vi "Day 23-Recurse Possible Moves.vi"(10 "Energy in":i32, 11 "State in":map{T1, T2[]}(c390)) -> (2 "Energy out":i32, 3 "State out":map{T1, T2[]}(c390))   [LabVIEW 2021]
uses:
  Amphipod Enum.ctl
  3c6be11d-fb2c-47dd-b0ed-e6924b9f2e6b.vi
  Zone Enum.ctl
  Hallway Positions Enum.ctl
  Room Enum.ctl
  Position Cluster.ctl
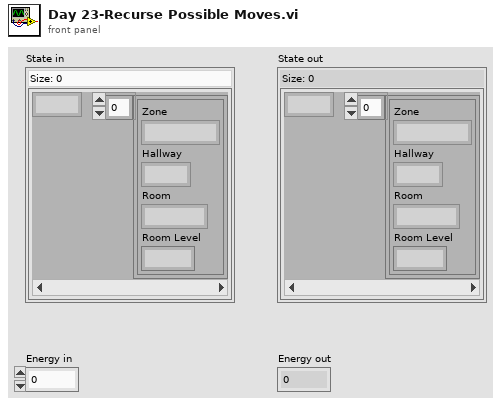
[diagram p1: front panel]
types:
  T1 = typedef "Amphipod Enum.ctl" = enum16{"A", "B", "C", "D"}
  T2 = typedef "Position Cluster.ctl" = cluster{"Zone":T3, "Hallway":T4, "Room":T5, "Room Level":i32}
  T3 = typedef "Zone Enum.ctl" = enum16{"Hallway", "Room"}
  T4 = typedef "Hallway Positions Enum.ctl" = enum16{"H1", "H2", "D3", "H4", "D5", "H6", "D7", "H8", "D9", "H10", "H11"}
  T5 = typedef "Room Enum.ctl" = enum16{"Room A", "Room B", "Room C", "Room D"}
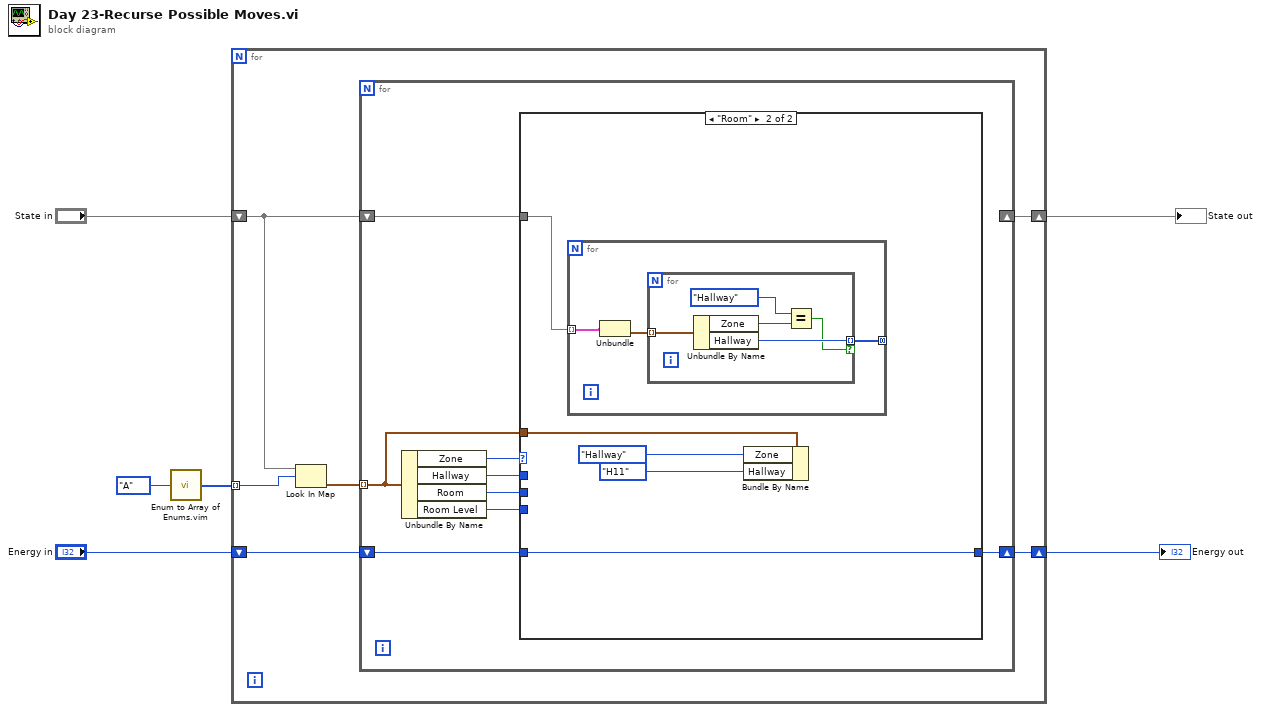
[diagram p0: block diagram]
diagram:
  n1 = call "Enum to Array of Enums.vim"("enum"=Amphipod_Enum."A" ("Amphipod Enum")) -> ("array of enums"=w1:T1[])
  n2 = for {
    tunnel: w1 -> [w12] mode=indexing
    shift-right: [w9] -> w6
    shift-left: "Energy in" -> [w10]
    shift-right: [w7] -> w3
    shift-left: "State in" -> [w8]
    n3 = Look In Map(map=w8, key=w12) -> (value=w11:T2[])  [unwired: 1 in, 1 out]
    n4 = for {
      tunnel: w11 -> [w13] mode=indexing
      shift-right: [w15] -> w9
      shift-left: w10 -> [w16]
      shift-right: [_] -> w7
      shift-left: w8 -> [w14]
      n5 = Unbundle By Name(w13) -> ("Zone"=w20:T3, "Hallway"=w19:T4, "Room"=w18:T5, "Room Level"=w17:i32)
      n6 = case shown="\"Room\"" w20 {
        tunnel: w19 -> [_ _]
        tunnel: w18 -> [_ _]
        tunnel: w17 -> [_ _]
        tunnel: w16 -> [w21 w26]
        tunnel: [w21 w26] -> w15
        tunnel: w14 -> [_ w22]
        tunnel: w13 -> [_ w25]
        frame "Hallway", Default {
        }
        frame "Room" {
          n7 = for {
            tunnel: w22 -> [w29] mode=indexing
            tunnel: [w27] -> _ mode=concatenating
            n8 = Unbundle(w29) -> (w28:T2[])  [unwired: 1 out]
            n9 = for {
              tunnel: w28 -> [w34] mode=indexing
              tunnel: [w33] -> w27 mode=indexing if=w30
              n10 = Unbundle By Name(w34) -> ("Zone"=w32:T3, "Hallway"=w33:T4)
              n11 = Equal?(x=Zone_Enum."Hallway", y=w32) -> (x = y?=w30:bool)
            }
          }
          n12 = Bundle By Name(cluster=w25, "Zone"=Zone_Enum."Hallway", "Hallway"=Hallway_Positions_Enum."H11") -> ()  [unwired: 1 out]
        }
      }
    }
  }
  "Energy out" <- w6
  "State out" <- w3
